vi "Actor Core.vi"(8 "error in":errorcluster, 11 "Nested in":refnum<class "NPad2.lvclass">) -> (0 "error out":errorcluster, 3 "Actor out":refnum<class "Actor.lvclass">)   [LabVIEW 2020, in "NPad2.lvlib" / "NPad2.lvclass"]
doc: "(<B>Filename</B>: Actor Framework.lvlib:Actor.lvclass:Actor Core.vi)\n\nReceives messages to the actor, reacts to them, and initiates any error handling that may shut the actor down.\n\nDescendant classes may override this VI to append parallel tasks for the actor to complete while it handles messages. Overrides use the Call Parent Method node."
uses:
  NPad2.lvclass
  C:/Program Files (x86)/National Instruments/LabVIEW 2020/vi.lib/ActorFramework/Actor/Actor.lvclass
  <vilib>/ActorFramework/Actor/Actor.lvclass
  <vilib>/ActorFramework/Actor/Actor.lvclass/Actor.ctl
  <vilib>/ActorFramework/Message Enqueuer/Message Enqueuer.lvclass/Message Enqueuer.ctl
  NPad2.lvclass/NPad2.ctl
  NPad2 Messages/Update_Event_number Msg/Update_Event_number Msg.lvclass/Update_Event_number Msg.ctl
  NPad2 Messages/Concatenate Msg/Concatenate Msg.lvclass/Concatenate Msg.ctl
  <vilib>/ActorFramework/Message Enqueuer/Init from Existing Queue.vi
  <vilib>/ActorFramework/Message Enqueuer/Enqueue.vi
  NPad2 Messages/Update_Event_number Msg/Update_Event_number Msg.lvclass
  C:/Program Files (x86)/National Instruments/LabVIEW 2020/vi.lib/ActorFramework/Message/Message.lvclass
  NPad2 Messages/OK Msg/OK Msg.lvclass
  NPad2 Messages/Concatenate Msg/Concatenate Msg.lvclass
  NPad2 Messages/minusOne Msg/minusOne Msg.lvclass
  NPad2 Messages/PlusOne Msg/PlusOne Msg.lvclass
  NPad2 Messages/BK Msg/BK Msg.lvclass
  <vilib>/ActorFramework/Stop Msg/Stop Msg.lvclass
  <vilib>/ActorFramework/Message Priority Queue/Priority Enqueue.vi
  <vilib>/ActorFramework/Message Enqueuer/Message Enqueuer.lvclass
panel:
  out "number":string
  in  "Npad":T1
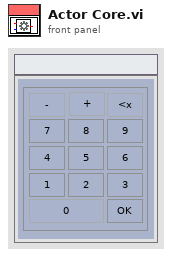
[diagram p1: front panel]
types:
  T1 = cluster{"3":bool, "2":bool, "1":bool, "6":bool, "5":bool, "4":bool, "9":bool, "8":bool, "7":bool, "OK":bool, "0":bool, "ba":bool, "-1":bool, "+1":bool}
  T2 = cluster{"Stop":refnum<user-event>, "number":refnum<user-event>}
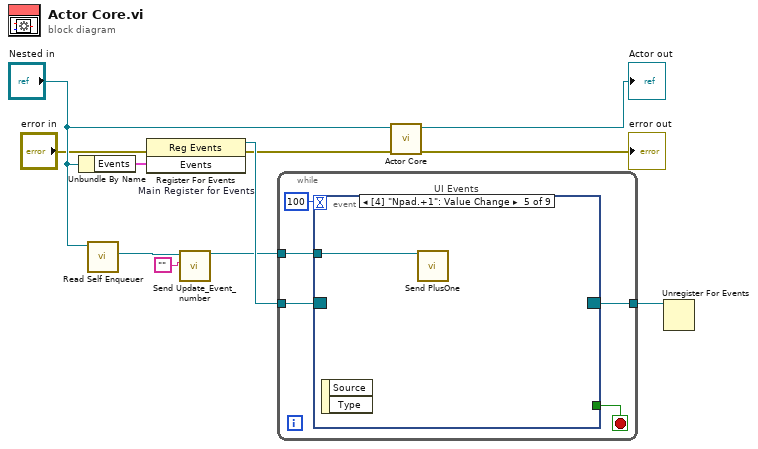
[diagram p0: block diagram]
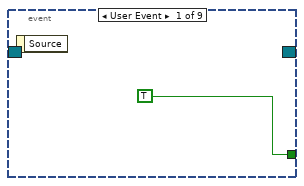
[diagram p2: hidden frame]
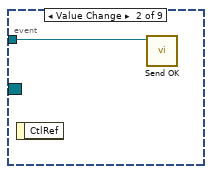
[diagram p3: hidden frame]
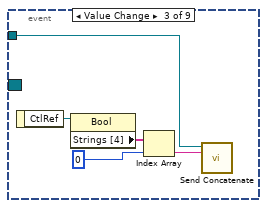
[diagram p4: hidden frame]
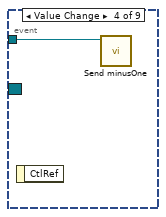
[diagram p5: hidden frame]
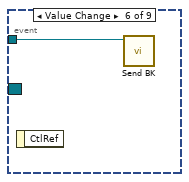
[diagram p6: hidden frame]
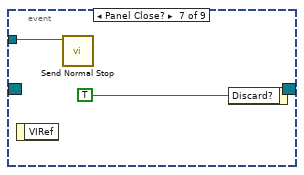
[diagram p7: hidden frame]
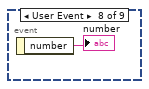
[diagram p8: hidden frame]
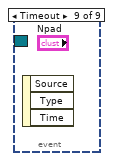
[diagram p9: hidden frame]
diagram:
  n1 = Unbundle By Name("Nested in") -> ("Events"=w8:T2)
  n2 = call <vilib>:"Read Self Enqueuer.vi"("Actor"="Nested in") -> ("Self Enqueuer"=w3:refnum<class "Message Enqueuer.lvclass">)  [unwired: 10 in]
  n3 = register-events "Main Register for Events"(error in="error in", w8) -> (reference out=w9:refnum<event-registration>, error out=w4:errorcluster)  [unwired: 1 in]
  n4 = call "Send Update_Event_number.vi"("number"="", "Message Enqueuer"=w3) -> ("Message Enqueuer out"=w2:refnum<class "Message Enqueuer.lvclass">)  [unwired: 8 in, 1 out]
  n5 = while {
    tunnel: w9 -> [w16]
    tunnel: [w14] -> w7
    tunnel: w2 -> [w13]
    stop <- w15 stop-if-true
    n6 = event "UI Events" shown="[4] \"Npad.+1\": Value Change" {
      selector: w16 -> [_ _ _ _ _ _ _ _ _]
      dyn-events: [_ _ _ _ _ _ _ _ _] -> w14
      timeout: 100 -> [_ _ _ _ _ _ _ _ _]
      tunnel: [TRUE _ _ _ _ _ _ _ _] -> w15
      tunnel: w13 -> [_ w18 w19 w24 w25 w26 w27 _ _]
      event User Event {
        n7 = event-data() -> ()  [unwired: 1 in, 1 out]
      }
      event "Npad.OK": Value Change {
        n8 = event-data() -> ()  [unwired: 1 in, 1 out]
        n9 = call "Send OK.vi"("Message Enqueuer"=w18) -> ()  [unwired: 9 in, 2 out]
      }
      event "Npad.1", "Npad.2", "Npad.3", "Npad.4", "Npad.5", "Npad.6", "Npad.7", "Npad.8", "Npad.9", "Npad.0": Value Change {
        n10 = event-data() -> ("CtlRef"=w23:refnum<vi>)  [unwired: 1 in]
        n11 = property class="Bool"(reference=w23) -> ("Strings [4]"=w22:string[])  [unwired: 1 in, 2 out]
        n12 = Index Array(array=w22, index=0) -> (element=w20:string)
        n13 = call "Send Concatenate.vi"("dataNpad"=w20, "Message Enqueuer"=w19) -> ()  [unwired: 8 in, 2 out]
      }
      event "Npad.-1": Value Change {
        n14 = event-data() -> ()  [unwired: 1 in, 1 out]
        n15 = call "Send minusOne.vi"("Message Enqueuer"=w24) -> ()  [unwired: 9 in, 2 out]
      }
      event "Npad.+1": Value Change {
        n16 = event-data() -> ()  [unwired: 1 in, 2 out]
        n17 = call "Send PlusOne.vi"("Message Enqueuer"=w25) -> ()  [unwired: 9 in, 2 out]
      }
      event "Npad.ba": Value Change {
        n18 = event-data() -> ()  [unwired: 1 in, 1 out]
        n19 = call "Send BK.vi"("Message Enqueuer"=w26) -> ()  [unwired: 9 in, 2 out]
      }
      event Panel Close? {
        n20 = event-data() -> ()  [unwired: 1 in, 1 out]
        n21 = call <vilib>:"Send Normal Stop.vi"("Message Enqueuer"=w27) -> ()  [unwired: 10 in, 1 out]
        n22 = event-data("Discard?"=TRUE) -> ()  [unwired: 1 in, 1 out]
      }
      event User Event {
        n23 = event-data() -> ("number"=→"number":string)  [unwired: 1 in]
      }
      event Timeout {
        n24 = event-data() -> ()  [unwired: 1 in, 3 out]
      }
    }
  }
  n25 = call-parent "Actor Core.vi"("error in"=w4, "Actor in"="Nested in") -> ("error out"=→"error out":errorcluster, "Actor out"=→"Actor out":refnum<class "Actor.lvclass">)  [unwired: 8 in]
  n26 = Unregister For Events(event registration refnum=w7) -> ()  [unwired: 1 in, 1 out]
